vi "theta2num-den-K.vi"(11 "theta":dbl[](array[numeric])) -> (1 "Den":dbl[](array[numeric]), 2 "Num":dbl[](array[numeric]), 3 "K":dbl)   [LabVIEW 2017]
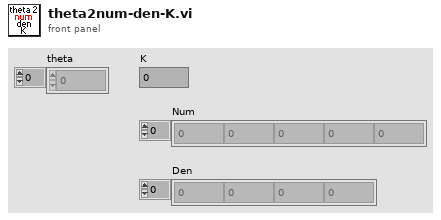
[diagram p1: front panel]
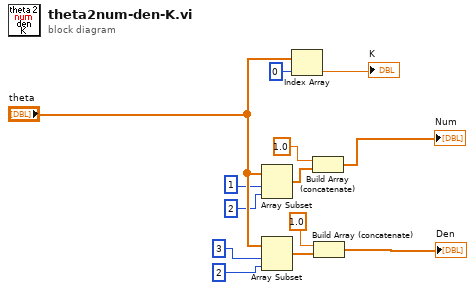
[diagram p0: block diagram]
diagram:
  n1 = Array Subset(array="theta", index=1, length=2 ("index")) -> (w7:dbl[])
  n2 = Array Subset(array="theta", index=3, length=2 ("index")) -> (w9:dbl[])
  n3 = Index Array(array="theta", index=0) -> (element=→"K":dbl)
  n4 = Build Array (concatenate)(1.0, w7) -> (→"Num":dbl[])
  n5 = Build Array (concatenate)(1.0, w9) -> (→"Den":dbl[])
